vi "raw_extract.vi"() -> ()   [LabVIEW 2012]
panel:
  out "Raw Image Data":string
  out "error out":errorcluster
  in  "error in":errorcluster
  in  "address":string="192.168.1.101"
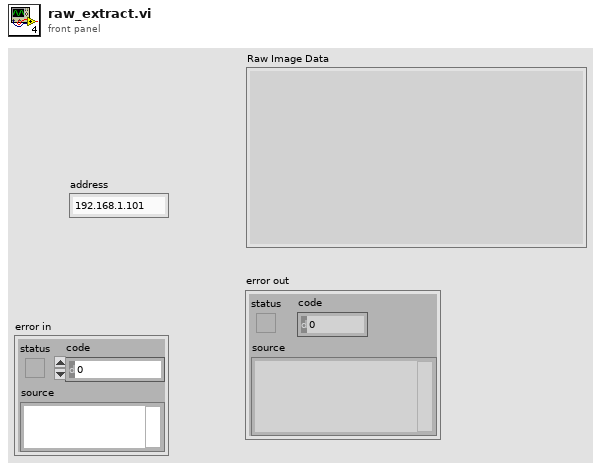
[diagram p1: front panel]
types:
  T1 = enum16{"Standard", "Buffered", "CRLF", "Immediate"}
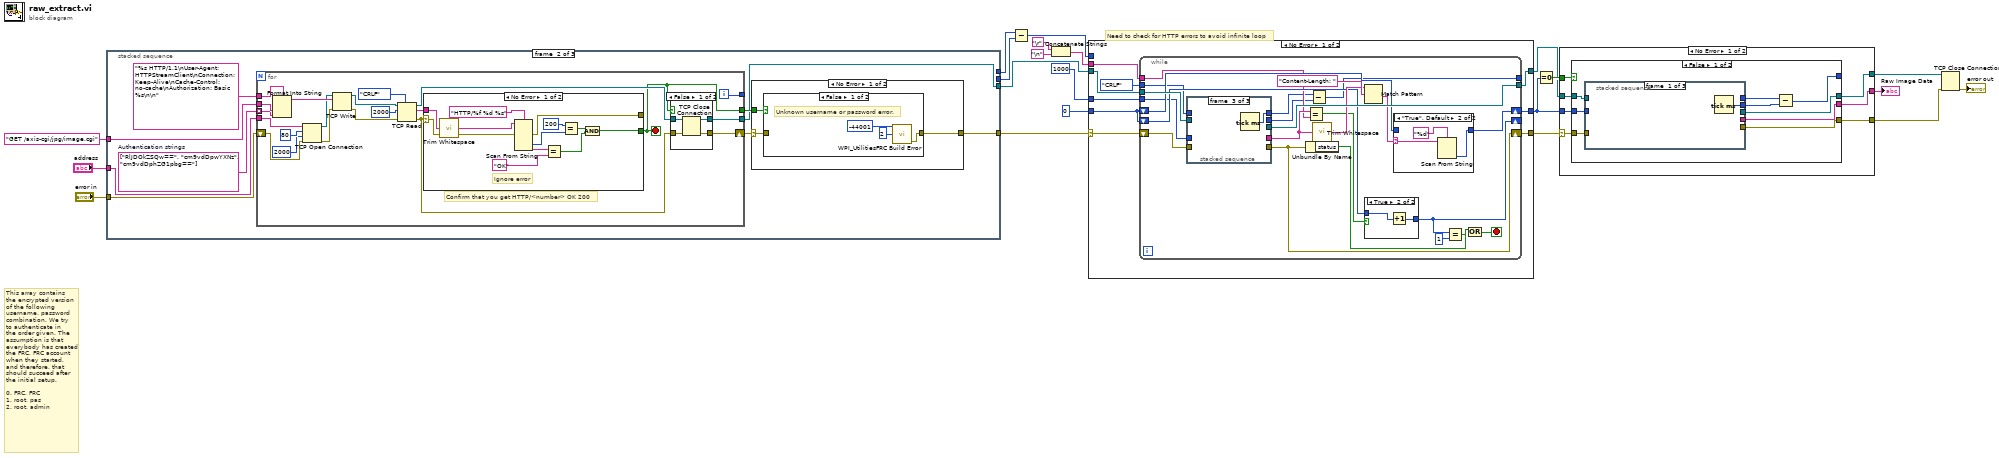
[diagram p0: block diagram]
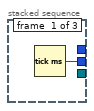
[diagram p2: hidden frame]
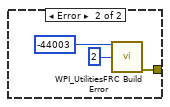
[diagram p4: hidden frame]
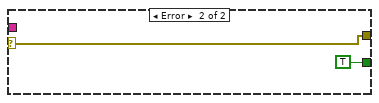
[diagram p6: hidden frame]
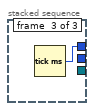
[diagram p7: hidden frame]
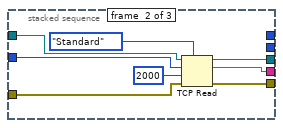
[diagram p8: hidden frame]
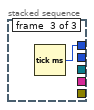
[diagram p9: hidden frame]
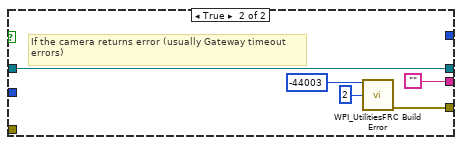
[diagram p10: hidden frame]
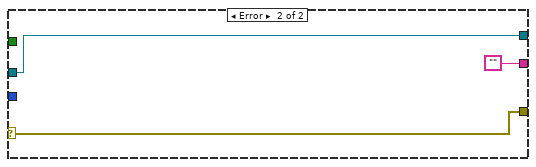
[diagram p11: hidden frame]
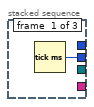
[diagram p12: hidden frame]
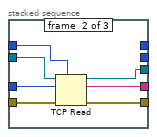
[diagram p13: hidden frame]
diagram:
  # "This array contains\nthe encrypted version\nof the following \nusername, password\ncombination. We try \nto authenticate in\nthe order given. The \nassumption is that \neverybody has created\nthe FRC, FRC account\nwhen they started,\nand therefore, that\nshould succeed after\nthe initial setup.\n\n0. FRC, FRC\n1. root, pas\n2. root, admin"
  # "Need to check for HTTP errors to avoid infinite loop"
  n1 = stacked-sequence {
    tunnel: "GET /axis-cgi/jpg/image.cgi" -> [_ w23 _]
    tunnel: [_ w27 _] -> w11
    tunnel: [_ w26 _] -> w10
    tunnel: "error in" -> [_ w25 _]
    tunnel: "address" -> [_ w24 _]
    tunnel: [w22 _ _] -> w3
    tunnel: [_ _ w83] -> w4
    frame #0 {
      n2 = Tick Count (ms)() -> (millisecond timer value=w22:u32)
    }
    frame #1 {
      w29 = string[] ["RlJDOkZSQw==", "cm9vdDpwYXNz", "cm9vdDphZG1pbg=="]  # Authentication strings
      n3 = for {
        shift-right: [w47] -> w30
        shift-left: w25 -> [w53]
        tunnel: "%s HTTP/1.1\nUser-Agent: HTTPStreamClient\nConnection: Keep-Alive\nCache-Control: no-cache\nAuthorization: Basic %s\n\n" -> [w58]
        tunnel: w23 -> [w57]
        tunnel: w29 -> [w56] mode=indexing
        tunnel: [w49] -> w31
        tunnel: [w48] -> w26
        tunnel: w24 -> [w46]
        tunnel: [w45] -> _
        i -> [w45]
        stop <- w49 stop-if-true
        # "Confirm that you get HTTP/<number> OK 200"
        n4 = Format Into String(format string=w58, w57, w56) -> (resulting string=w55:string)  [unwired: 2 in, 1 out]
        n5 = TCP Open Connection(address=w46, remote port or service name=u16 80, timeout ms (60000)=2000, error in (no error)=w53) -> (connection ID=w54:refnum<k5>, error out=w52:errorcluster)  [unwired: 1 out]
        n6 = TCP Write(connection ID=w54, data in=w55, error in (no error)=w52) -> (connection ID out=w60:refnum<k5>, error out=w59:errorcluster)  [unwired: 2 out]
        n7 = TCP Read(connection ID=w60, bytes to read=2000, error in (no error)=w59, 7:T1."CRLF" ("mode (standard)")) -> (connection ID out=w51:refnum<k5>, data out=w42:string, error out=w50:errorcluster)  [unwired: 1 out]
        n8 = case shown="No Error" w50 {
          selector: w50 -> [w72 w82]
          tunnel: [w73 TRUE] -> w49
          tunnel: [w71 w82] -> _
          tunnel: w42 -> [w69 _]
          frame No Error {
            # "Ignore error"
            n9 = call <vilib>:"Trim Whitespace.vi"("string"=w69) -> ("trimmed string"=w70:string)  [unwired: 1 in]
            n10 = Scan From String(format string="HTTP/%f %d %s", input string=w70, error in=w72) -> (error out=w71:errorcluster, output 2=w79:i32, output 3=w77:string)  [unwired: 1 in, 6 out]
            n11 = Equal?(x=w77, y="OK" ("format string")) -> (x = y?=w75:bool)
            n12 = Equal?(x=200, y=w79) -> (x = y?=w74:bool)
            n13 = And(x=w74, y=w75) -> (x .and. y?=w73:bool)
          }
          frame Error {
          }
        }
        n14 = case shown="False" w49 {
          tunnel: w51 -> [w66 w68]
          tunnel: w50 -> [w65 w67]
          tunnel: [w64 w68] -> w48
          tunnel: [w63 w67] -> w47
          frame False {
            n15 = TCP Close Connection(connection ID=w66, error in (no error)=w65) -> (connection ID out=w64:refnum<k5>, error out=w63:errorcluster)  [unwired: 1 out]
          }
          frame True {
          }
        }
      }
      n16 = case shown="No Error" w30 {
        selector: w30 -> [w32 _]
        tunnel: w31 -> [w34 _]
        tunnel: [w33 w39] -> w27
        frame No Error {
          n17 = case shown="False" w34 {
            tunnel: [w35 w38] -> w33
            tunnel: w32 -> [_ w38]
            frame False {
              # "Unknown username or password error."
              n18 = call <vilib>:"WPI_UtilitiesFRC Build Error.vi"("error code"=-44001 ("code"), "chain levels to remove (1)"=2) -> ("error out"=w35:errorcluster)  [unwired: 3 in, 10 out]
            }
            frame True {
            }
          }
        }
        frame Error {
          n19 = call <vilib>:"WPI_UtilitiesFRC Build Error.vi"("error code"=-44003 ("code"), "chain levels to remove (1)"=2) -> ("error out"=w39:errorcluster)  [unwired: 3 in, 10 out]
        }
      }
    }
    frame #2 {
      n20 = Tick Count (ms)() -> (millisecond timer value=w83:u32)
    }
  }
  n21 = Subtract(x=w4, y=w3) -> (x-y=w2:u32)
  n22 = Concatenate Strings("\r", "\n") -> (w17:string)
  n23 = case shown="No Error" w11 {
    selector: w11 -> [w84 w132]
    tunnel: [w92 w132] -> w8
    tunnel: [w91 w133] -> w13
    tunnel: [w90 w134] -> w12
    tunnel: w17 -> [w89 _]
    tunnel: 0 -> [w88 w133]
    tunnel: w10 -> [w86 w134]
    tunnel: 1000 ("bytes to read") -> [w85 _]
    tunnel: w2 -> [_ _]
    frame No Error {
      n24 = while {
        tunnel: w86 -> [w115]
        tunnel: [w114] -> w90
        shift-right: [w110] -> w91
        shift-left: w88 -> [w109]
        shift-right: [w106] -> _
        shift-left: w88 -> [w107]
        tunnel: w89 -> [w103]
        tunnel: w85 -> [w102]
        tunnel: T1."CRLF" ("mode (standard)") -> [w101]
        shift-right: [w99] -> w92
        shift-left: w84 -> [w100]
        tunnel: [w93] -> _
        stop <- w96 stop-if-true
        n25 = stacked-sequence {
          tunnel: w115 -> [_ w123 _]
          tunnel: [_ w122 _] -> w114
          tunnel: [_ w121 _] -> w104
          tunnel: w102 -> [_ w120 _]
          tunnel: w101 -> [_ w119 _]
          tunnel: w100 -> [_ w118 _]
          tunnel: [_ w117 _] -> w99
          tunnel: [w116 _ _] -> w94
          tunnel: [_ _ w124] -> w95
          frame #0 {
            n26 = Tick Count (ms)() -> (millisecond timer value=w116:u32)
          }
          frame #1 {
            n27 = TCP Read(connection ID=w123, bytes to read=w120, error in (no error)=w118, 7:w119) -> (connection ID out=w122:refnum<k5>, data out=w121:string, error out=w117:errorcluster)  [unwired: 1 out]
          }
          frame #2 {
            n28 = Tick Count (ms)() -> (millisecond timer value=w124:u32)
          }
        }
        n29 = Unbundle By Name(w99) -> ("status"=w98:bool)
        n30 = Equal?(x=w104, y=w103) -> (x = y?=w108:bool)
        n31 = Subtract(x=w95, y=w94) -> (x-y=w93:u32)
        n32 = call <vilib>:"Trim Whitespace.vi"("string"=w104) -> ("trimmed string"=w112:string)  [unwired: 1 in]
        n33 = Match Pattern(string=w112, regular expression="Content-Length: ") -> (after substring=w111:string)  [unwired: 4 out]
        n34 = case shown="True" w108 {
          tunnel: w107 -> [w125 w127]
          tunnel: [w125 w126] -> w106
          frame False {
          }
          frame True {
            n35 = Increment(x=w127) -> (x+1=w126:i32)
          }
        }
        n36 = case shown="\"True\", Default" w111 {
          selector: w111 -> [_ w130]
          tunnel: [w128 w131] -> w110
          tunnel: w109 -> [w128 _]
          frame "" {
          }
          frame "True", Default {
            n37 = Scan From String(format string="%d", input string=w130) -> (output 1=w131:i32)  [unwired: 2 in, 4 out]
          }
        }
        n38 = Equal?(x=w106, y=1) -> (x = y?=w97:bool)
        n39 = Or(x=w98, y=w97) -> (x .or. y?=w96:bool)
      }
    }
    frame Error {
    }
  }
  n40 = Equal To 0?(x=w13) -> (x = 0?=w14:bool)
  n41 = case shown="No Error" w8 {
    selector: w8 -> [w135 w168]
    tunnel: [w141 w168] -> w21
    tunnel: [w140 ""] -> w20
    tunnel: [w139 w166] -> w15
    tunnel: w14 -> [w138 _]
    tunnel: w13 -> [w137 _]
    tunnel: w12 -> [w136 w166]
    frame No Error {
      n42 = case shown="False" w138 {
        tunnel: w136 -> [w150 w164]
        tunnel: [w149 w161] -> w141
        tunnel: [w147 ""] -> w140
        tunnel: w137 -> [w148 _]
        tunnel: [w146 w164] -> w139
        tunnel: w135 -> [w145 _]
        tunnel: [w142 _] -> _
        frame False {
          n43 = stacked-sequence {
            tunnel: w150 -> [_ w159 _]
            tunnel: [_ w158 _] -> w149
            tunnel: w148 -> [_ w155 _]
            tunnel: [_ w154 _] -> w147
            tunnel: [_ w153 _] -> w146
            tunnel: w145 -> [_ w152 _]
            tunnel: [_ _ w160] -> w144
            tunnel: [w151 _ _] -> w143
            frame #0 {
              n44 = Tick Count (ms)() -> (millisecond timer value=w151:u32)
            }
            frame #1 {
              n45 = TCP Read(connection ID=w159, bytes to read=w155, error in (no error)=w152, 7:T1."Standard" ("mode (standard)"), 9:2000 ("timeout ms (25000)")) -> (connection ID out=w153:refnum<k5>, data out=w154:string, error out=w158:errorcluster)
            }
            frame #2 {
              n46 = Tick Count (ms)() -> (millisecond timer value=w160:u32)
            }
          }
          n47 = Subtract(x=w144, y=w143) -> (x-y=w142:u32)
        }
        frame True {
          # "If the camera returns error (usually Gateway timeout\nerrors)"
          n48 = call <vilib>:"WPI_UtilitiesFRC Build Error.vi"("error code"=-44003 ("code"), "chain levels to remove (1)"=2) -> ("error out"=w161:errorcluster)  [unwired: 3 in, 10 out]
        }
      }
    }
    frame Error {
    }
  }
  "Raw Image Data" <- w20
  n49 = TCP Close Connection(connection ID=w15, error in (no error)=w21) -> (error out=→"error out":errorcluster)  [unwired: 2 out]
